vi "dms-main-train-2.vi"() -> ()   [LabVIEW 2015]
uses:
  states-enum.ctl
  <vilib>/platform/TimedLoop/XDataNode/XDataNode.xnode
  <vilib>/Platform/TimedLoop/XDataNode/nitl_modes.ctl
  <vilib>/Platform/TimedLoop/XDataNode/XDNodeRunTimeDep.lvlib
  <vilib>/Platform/TimedLoop/XDataNode/wakeup.ctl
  <vilib>/Platform/TimedLoop/XDataNode/timing_clust.ctl
  Device/Methods/Speaker-Play.vi
  Rack/Methods/Rack-Refresh.vi
  Device/Methods/Lickometer-Read.vi
  Device/Methods/Valve-Init.vi
  Device/Methods/Juicer-Init.vi
  Device/Methods/Speaker-Init.vi
  Rack/Methods/Rack-Start.vi
  Rack/Methods/Rack-Config.vi
  Device/Methods/Lickometer-Init.vi
  Rack/Methods/Rack-Init.vi
  Device/Methods/Valve-Pulse.vi
  <vilib>/Utility/file.llb/Read Delimited Spreadsheet (I64).vi
  Device/Methods/Lickometer-Stop.vi
  Rack/Methods/Rack-Stop.vi
  Rack/Typedefs/OutputRequest.ctl
  Rack/Typedefs/OutputRequest refnum.ctl
  Rack/Methods/Port drivers/DigitalInput-DataCluster.ctl
  Rack/Typedefs/InputData cluster.ctl
  Device/Typedefs/Lickometer.ctl
  Device/Typedefs/Speaker.ctl
  Device/Typedefs/Juicer.ctl
  Device/Typedefs/Valve.ctl
panel:
  out "InputData 3":T1
  out "InputData 2":T1
  in  "stop":bool
  out "Acc":dbl
  out "Time":dbl format="%#.0f"
  out "Trials":string
  out "Reward Dispensed (uL)":string
  out "Licks":string
  out "CR":string
  out "Miss":string
  out "FA":string
  out "Hits":string
  out "Current State":string
  out "Time Elapsed":dbl format="%<%H:%M:%S>t"
  in  "Tab Control":enum32{"Required", "Optional", "Devices"}(tab)
  in  "Tone Pairs":u16(ring) items=["1: 3000 Hz, 12000 Hz", "2: 5800 Hz, 5000 Hz", "3: 5000 Hz, 10000 Hz", "4: 8000 Hz, 15000 Hz"]
  in  "Max Time (s)":dbl=3600.0
  in  "Number of trials":string(combo)="500"
  in  "Max number of \nconsecutive trials":string(combo)="3"
  in  "Animal Name":string="Mouse"
  in  "Reward Vol. (uL)":dbl=5.0
  in  "Sequence Directory":path=path "C:/Users/SiapasLab/Desktop/git/wheatley"
  in  "Assay Description":string="Auditory delayed match to sample"
  in  "Recording Location":string="BI Room 146"
  in  "Trial delay (ms)":dbl=1500.0
  in  "Punish Time (s)":dbl
  in  "Trial window (ms)":dbl=1000.0
  in  "ITI lower (s)":dbl=10.0
  in  "ITI upper (s)":dbl=10.0
  in  "Min Licks":i32=1 min=1
  in  "Data Saving Directory":path=path "\\\\CA1-17\\ld8007/anesthesia/data"
  in  "Lickometer":T3={"Settings"={"Min lick duration"=1, "Port name"="bnc_panel.p0.3", "Port index"=0}, "Lick"=FALSE, "Debouncing"={"Semaphore"=refnum, "Lick start"=0}, "OutputRequest event ref"=refnum, "InputData reference"=refnum, "Active hi?"=FALSE}
  out "InputData":T1
  in  "Speaker":T6={"Settings"={"Portname"="BNC_Panel.ao0", "Index"=0, "Timestamp portname"="BNC_Panel.P0.0"}, "OutputRequest event ref"=refnum, "InputData reference"=refnum}
  in  "Juicer":T7={"Mode"=enum."Juice/reward", "Settings"={"Bleed #1 port index"=1, "Bleed #1 port name"="juicer.bleed1", "Bleed #2 port name"="juicer.bleed2", "Bleed #2 port index"=2, "Flush port name"="juicer.flush", "Flush port index"=3, "Purge port name"="juicer.purge", "Purge port index"=0, "Timestamp port name"="dsub_panel.p9.7"}, "OutputRequest event ref"=refnum, "InputData reference"=refnum}
  in  "Valve":T8={"Settings"={"Timestamp port name"="BNC_panel.P0.0", "Port name"="BNC_panel.P0.1", "Port index"=4}, "OutputRequest event ref"=refnum, "InputData reference"=refnum, "Default length (ms)"=100}
  # "Auditory delayed match to sample task (DMS)"
  # "(must be on same NI card)"
  # "(must be on same NI card)"
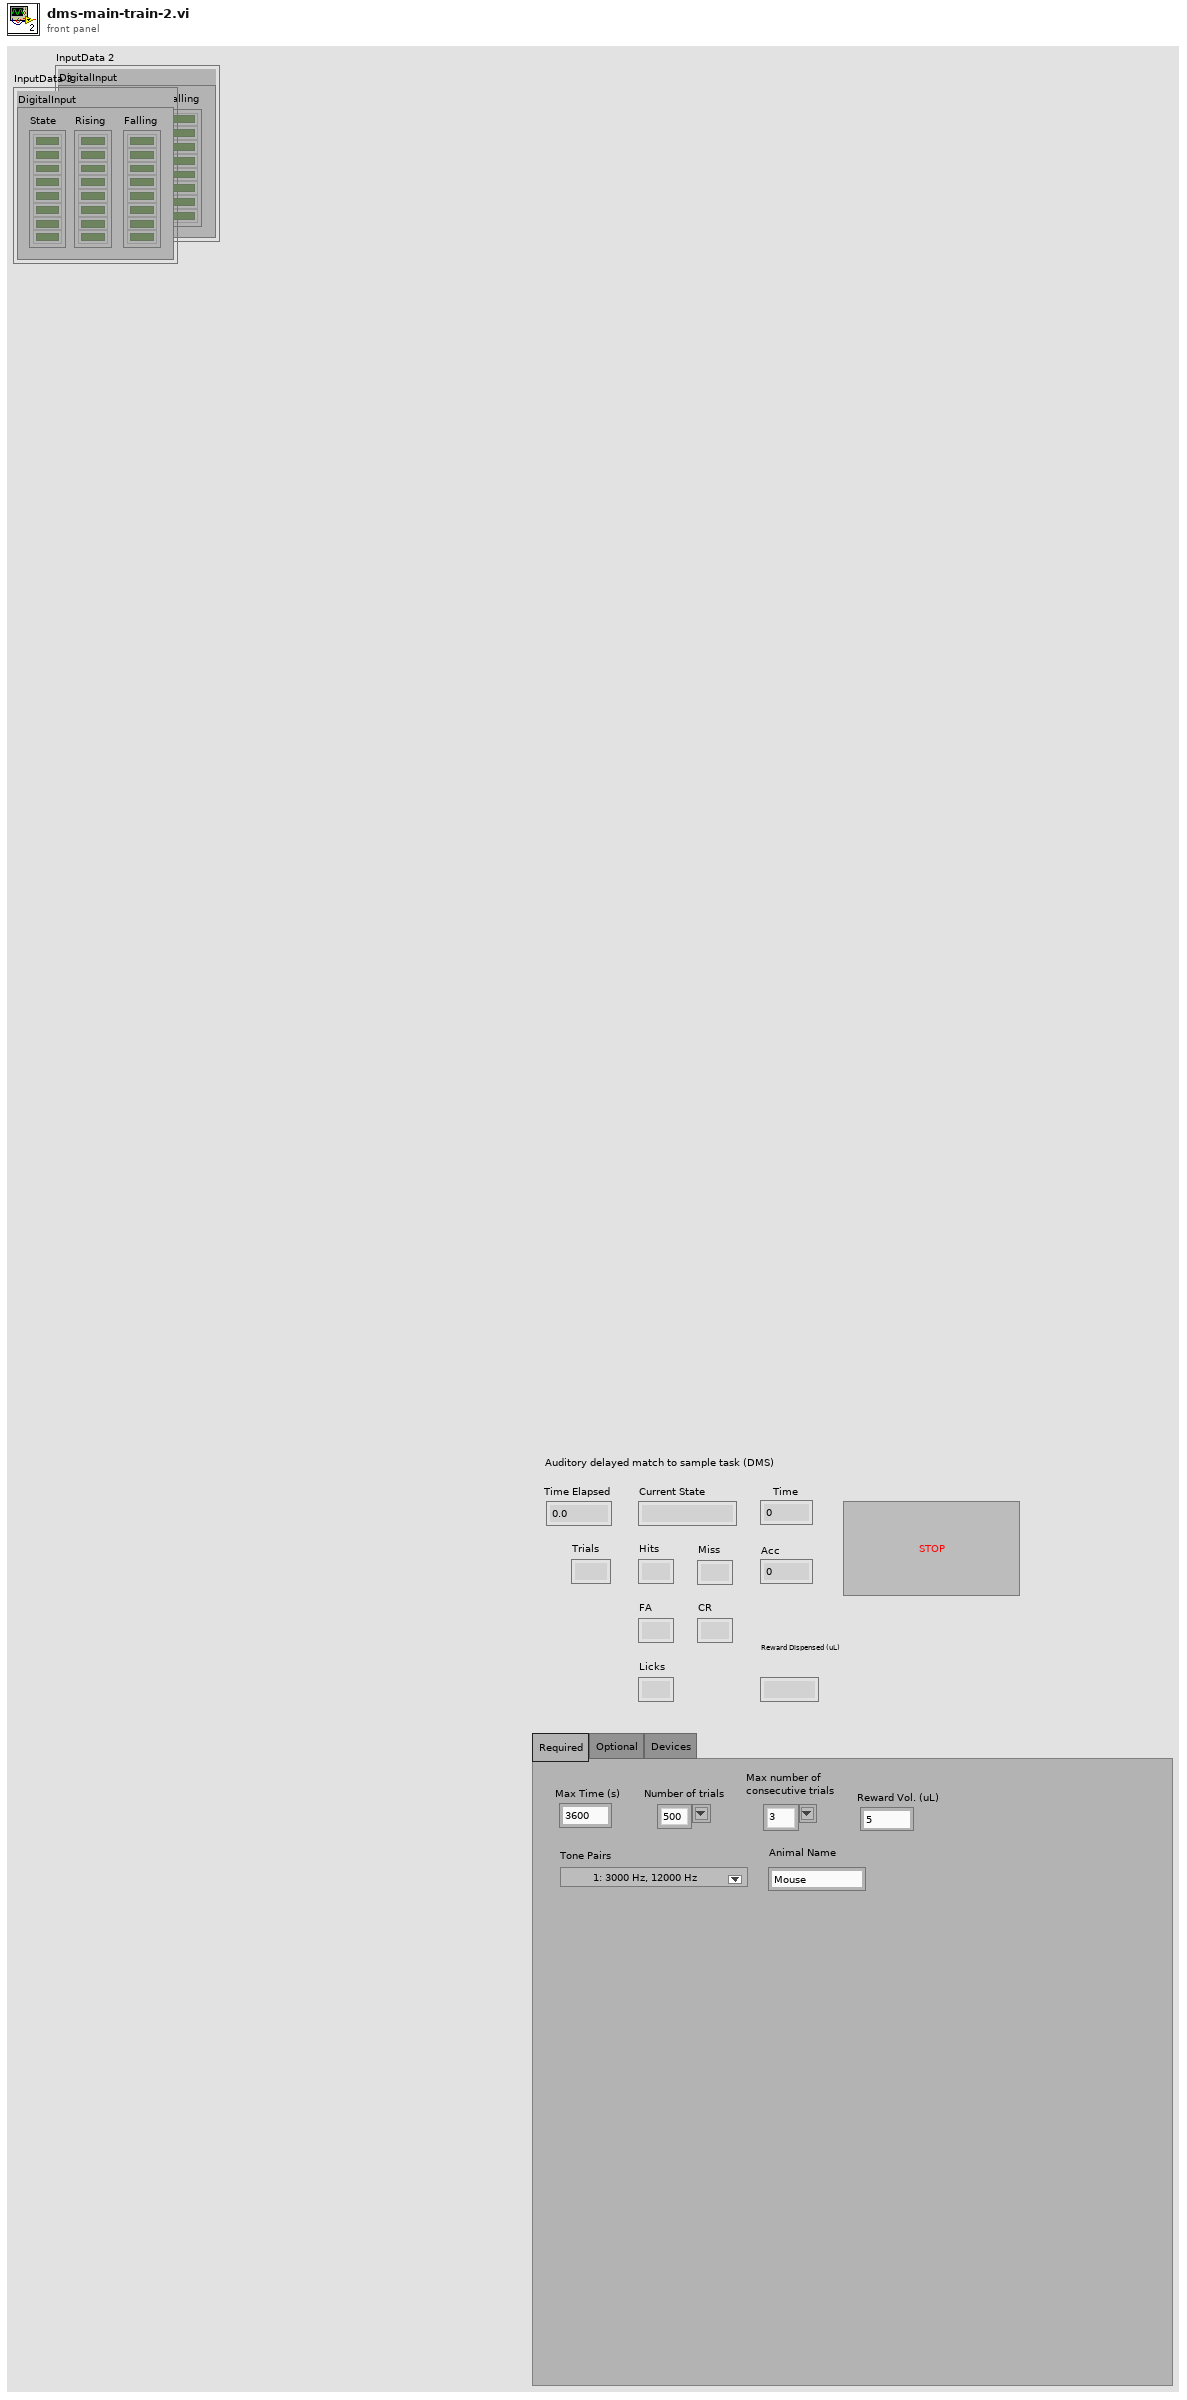
[diagram p1: front panel]
types:
  T1 = typedef "InputData cluster.ctl" = cluster{"DigitalInput":T2}
  T2 = typedef "DigitalInput-DataCluster.ctl" = cluster{"Falling":bool[], "Rising":bool[], "State":bool[]}
  T3 = typedef "Lickometer.ctl" = cluster{"Settings":cluster{"Min lick duration":u32, "Port name":string, "Port index":i32}, "Lick":bool, "Debouncing":cluster{"Semaphore":T4, "Lick start":u32}, "OutputRequest event ref":T5, "InputData reference":refnum<vi>, "Active hi?":bool}
  T4 = typedef "Semaphore RefNum" = refnum<k1>
  T5 = typedef "OutputRequest refnum.ctl" = refnum<user-event>
  T6 = typedef "Speaker.ctl" = cluster{"Settings":cluster{"Portname":string, "Index":i32, "Timestamp portname":string}, "OutputRequest event ref":T5, "InputData reference":refnum<vi>}
  T7 = typedef "Juicer.ctl" = cluster{"Mode":enum16{"Off", "Juice/reward", "Water flush", "Air purge"}, "Settings":cluster{"Bleed #1 port index":i32, "Bleed #1 port name":string, "Bleed #2 port name":string, "Bleed #2 port index":i32, "Flush port name":string, "Flush port index":i32, "Purge port name":string, "Purge port index":i32, "Timestamp port name":string}, "OutputRequest event ref":T5, "InputData reference":refnum<vi>}
  T8 = typedef "Valve.ctl" = cluster{"Settings":cluster{"Timestamp port name":string, "Port name":string, "Port index":i32}, "OutputRequest event ref":T5, "InputData reference":refnum<vi>, "Default length (ms)":i32}
  T9 = typedef "states-enum.ctl" = enum16{"ITI", "Trial", "Stop"}
  T10 = typedef "Rack driver configuration cluster.ctl" = cluster{"DigitalInput":T11, "DigitalOutput":T12, "FileOutput":T13, "AnalogOutput":T14, "DataSocketOutput":T15}
  T11 = typedef "DigitalInput-Configuration.ctl" = cluster{"Lines":tag[], "Refresh period (ms)":u32}
  T12 = typedef "DigitalOutput-Configuration.ctl" = cluster{"Output Lines":tag[], "DO timestamp lines":tag[], "Timestamp lines":tag[]}
  T13 = typedef "FileOutput-Configuration.ctl" = cluster{"Logfile path":path}
  T14 = typedef "AnalogOutput-Configuration.ctl" = cluster{"Output Lines":tag[], "AO timestamp lines":tag[]}
  T15 = typedef "DataSocketOutput-Configuration.ctl" = cluster{"DataSocket URL":string}
  T16 = cluster{"ITI upper (s)":dbl, "ITI lower (s)":dbl, "Punish Time (s)":dbl, "Trial window (ms)":dbl, "Trial delay (ms)":dbl, "Max Time (s)":dbl, "Min Licks":i32, "Reward Vol. (uL)":dbl, "Tone 1":i32, "Tone 2":i32}
  T17 = cluster{"appended path":path, "relative seconds":dbl, "Current Trial Index":i32, "Accuracy":dbl, "Hits":i32, "Miss":i32, "False Alarm":i32, "Correct Rejection":i32, "Licks":i32, "Reward Dispensed":dbl, "Punish ITI":bool, "Next Trial":i32}
  T18 = typedef "XDNodeRunTimeDep.lvlib/timing_clust.ctl" = cluster{"Expected End [f-1]":u64, "Actual End [f-1]":u64, "Finished Late? [f-1]":bool, "Expected End [i-1]":u64, "Actual End [i-1]":u64, "Finished Late? [i-1]":bool, "Expected Start [i]":u64, "Actual Start [i]":u64, "Expected Start [f]":u64, "Actual Start [f]":u64, "Source Name":string, "Structure Name":string, "Period":i64, "Deadline":i64, "Offset":i64, "Start":i64, "Priority":i32, "Timeout":i32, "Mode":T19, "Wakeup Reason":T20, "Error":errorcluster, "Source Type":string, "Secondary Source Type":string, "Global End Time":u64, "Global Start Time":u64, "Frame Duration":u64, "Iteration Duration":u64, "Assigned CPU":i32, "I/O Scan Engine Mode":u32}
  T19 = typedef "XDNodeRunTimeDep.lvlib/nitl_modes.ctl" = enum32{"No Change", "Process missed periods, maintain original phase", "Discard missed periods, maintain original phase", "Process missed periods, ignore original phase", "Discard missed periods, ignore original phase"}
  T20 = typedef "XDNodeRunTimeDep.lvlib/wakeup.ctl" = enum32{"Normal", "Aborted", "Asynchronous wakeup", "Timing source error", "Timed loop error", "Timeout"}
  T21 = cluster{"Trial Hit":bool, "Trial Miss":bool, "Trial FA":bool, "Trial CR":bool, "Skip Receiving":bool}
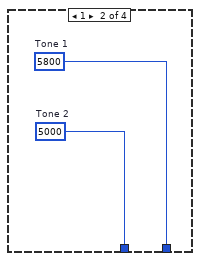
[diagram p2: hidden frame]
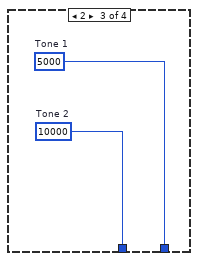
[diagram p3: hidden frame]
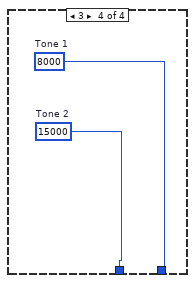
[diagram p4: hidden frame]
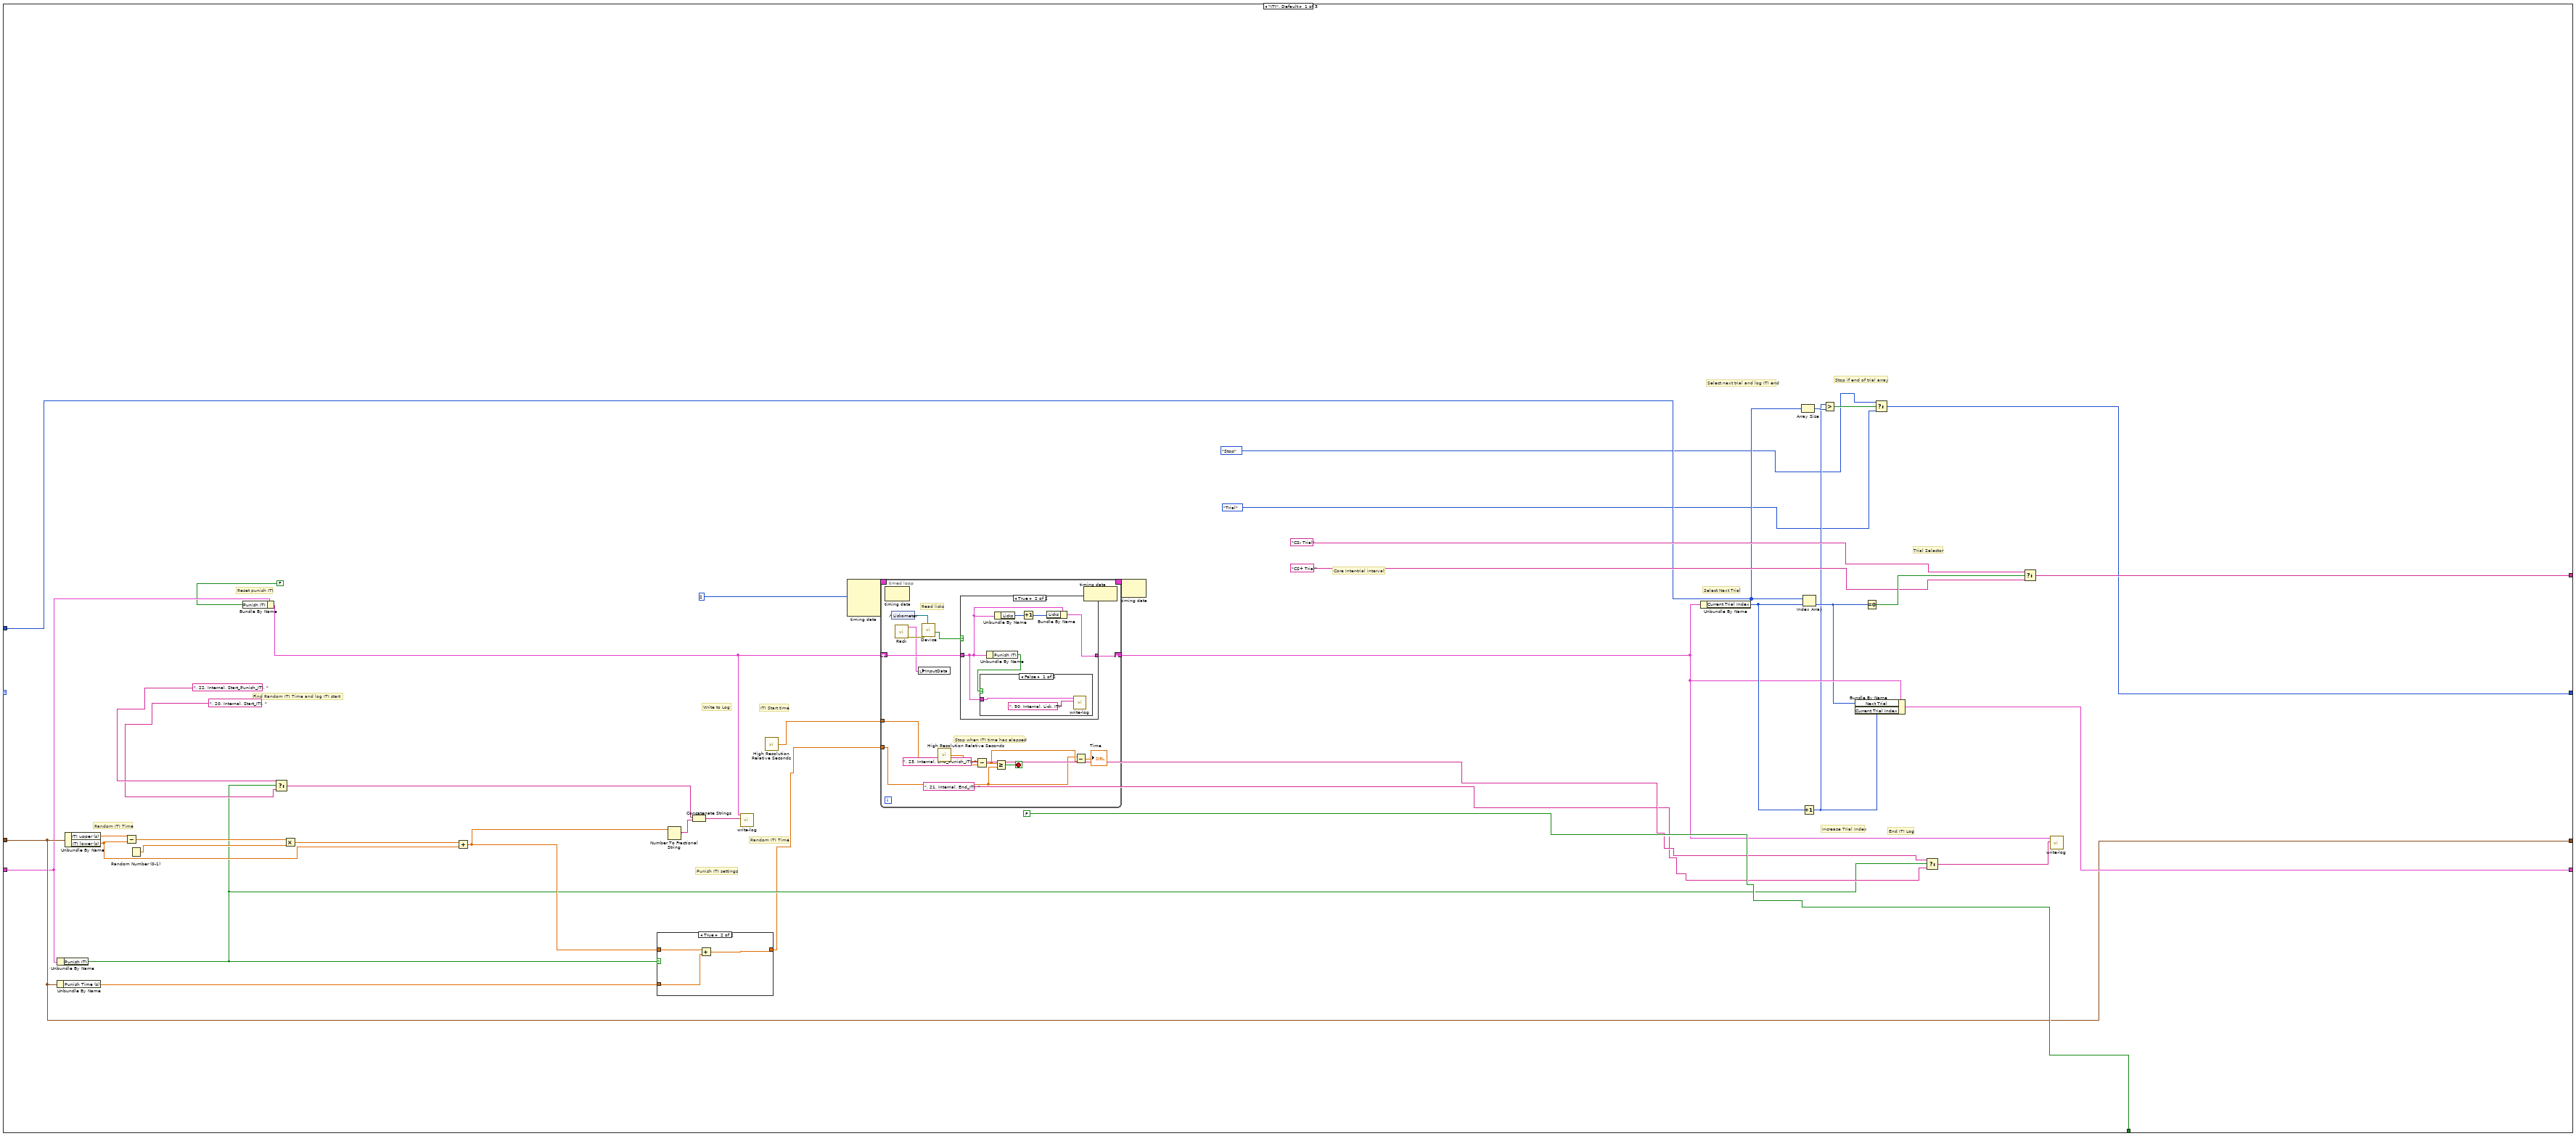
[diagram p6: hidden frame]
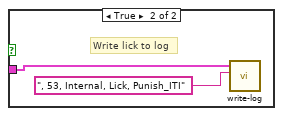
[diagram p8: hidden frame]
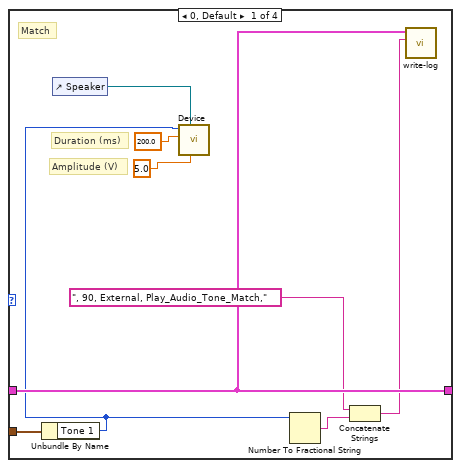
[diagram p11: hidden frame]
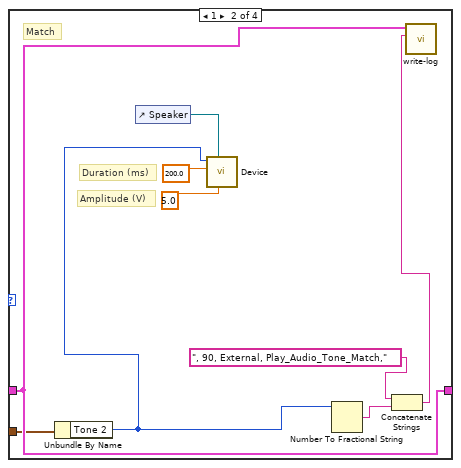
[diagram p12: hidden frame]
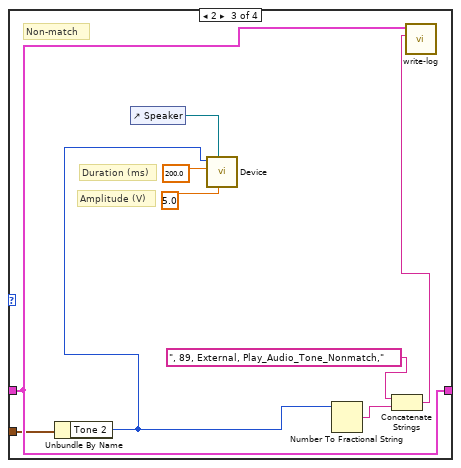
[diagram p13: hidden frame]
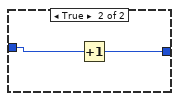
[diagram p14: hidden frame]
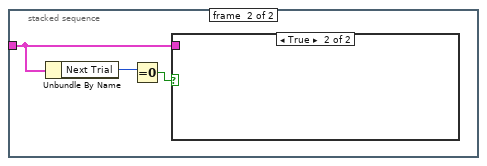
[diagram p16: hidden frame]
diagram:
  w141 = 0  # Next Trial
  w142 = FALSE  # Punish ITI
  w151 = 0.0  # Reward Dispensed
  w152 = 0  # Licks
  w153 = 0  # Correct Rejection
  w154 = 0  # False Alarm
  w157 = 0.0  # Accuracy
  w155 = 0  # Miss
  w156 = 0  # Hits
  w158 = 0  # Current Trial Index
  # "Create directory"
  # "Lickometer"
  # "Lickometer"
  # "Devices"
  # "Tone Pair Interpretation"
  # "Exit Logging"
  # "Front Panel Logging"
  # "CS+\nDelay lick: Miss\nReception lick: Hit\nNo lick: Miss\n\nCS-\nDelay lick: False alarm\nReception lick: False alarm\nNo lick: Correct reject"
  # "Start time"
  # "Internal Variables"
  # "External variables from Front Panel"
  # "External variable cluster"
  # "Internal variable cluster"
  # "State enum"
  # "Trial shift register"
  # "State machine"
  # "Front Panel Elements"
  # "Write trial sequence to log"
  # "Human readable time"
  # "End of header delimiter"
  # "Start Time"
  # "Environment"
  # "Schedule"
  # "Initialize data logger"
  # "Random sequence selection"
  # "Read in entire .csv"
  # "Load pre-generated sequences"
  n1 = Format Date/Time String(time format string (%c)="%Y-%m-%d-%H-%M-%S") -> (date/time string=w4:string)  [unwired: 2 in]
  n2 = case shown="0, Default" "Tone Pairs" {
    tunnel: [w224 w225 w227 w229] -> w39
    tunnel: [w223 w226 w228 w230] -> w40
    frame 0, Default {
      w224 = 12000  # Tone 2
      w223 = 3000  # Tone 1
    }
    frame 1 {
      w225 = 5000  # Tone 2
      w226 = 5800  # Tone 1
    }
    frame 2 {
      w227 = 10000  # Tone 2
      w228 = 5000  # Tone 1
    }
    frame 3 {
      w229 = 15000  # Tone 2
      w230 = 8000  # Tone 1
    }
  }
  n3 = Build Path(base path="Data Saving Directory", name or relative path=w4) -> (appended path=w2:path)
  n4 = Create Folder(path (use dialog)=w2) -> (created path=w1:path)  [unwired: 2 in, 2 out]
  n5 = control-ref of="InputData"() -> (w13:refnum<vi>)
  n6 = Build Path(base path=w1, name or relative path="data.txt") -> (appended path=w148:path)
  n7 = call-poly "Rack.vi"() -> ("error out"=w7:errorcluster, "OutputRequest\nevent ref"=w8:T5)  [unwired: 10 in]
  n8 = control-ref of="Juicer"() -> (w6:refnum<vi>)
  n9 = Path To String(path="Sequence Directory") -> (string=w96:string)
  n10 = call-poly "Device.vi"("Device reference"=w6, "error in (no error)"=w7, "OutputRequest event ref"=w8, "InputData reference"=w13) -> ("error out"=w10:errorcluster, "OutputRequest (dup)"=w15:T5, "InputData (dup)"=w12:refnum<vi>)  [unwired: 5 in]
  n11 = control-ref of="Valve"() -> (w5:refnum<vi>)
  n12 = Concatenate Strings(w96, "\\sequences\\seq_n_", "Number of trials", "_k_" ("string"), "Max number of \nconsecutive trials", "_m_2.csv" ("string")) -> (w214:string)
  n13 = call-poly "Device.vi"("Device reference"=w5, "error in (no error)"=w10, "OutputRequest event ref"=w15, "InputData reference"=w12) -> ("error out"=w9:errorcluster, "OutputRequest (dup)"=w14:T5, "InputData (dup)"=w11:refnum<vi>)  [unwired: 5 in]
  n14 = String To Path(string=w214) -> (path=w215:path)
  n15 = control-ref of="Speaker"() -> (w16:refnum<vi>)
  n16 = Concatenate Strings("Schedule," ("string"), "Assay Description", "\r\n") -> (w205:string)
  n17 = call-poly "Device.vi"("Device reference"=w16, "error in (no error)"=w9, "OutputRequest event ref"=w14, "InputData reference"=w11) -> ("error out"=w18:errorcluster, "OutputRequest (dup)"=w19:T5, "InputData (dup)"=w17:refnum<vi>)  [unwired: 5 in]
  n18 = Concatenate Strings("Path," ("string"), w96, "\r\n") -> (w99:string)
  n19 = call-poly <vilib>:"Read Delimited Spreadsheet.vi"("file path (dialog if empty)"=w215, "number of rows (all:-1)"=-1, "delimiter (\\t)"="," ("delimiter (\\t)")) -> ("all rows"=w209:i64[][])  [unwired: 7 in, 5 out]
  n20 = Write to Text File(file (use dialog)=w148, text=w205) -> (refnum out=w207:refnum<file>)  [unwired: 2 in, 2 out]
  n21 = control-ref of="Lickometer"() -> (w23:refnum<vi>)
  n22 = call-poly "Device.vi"("Device reference"=w23, "error in (no error)"=w18, "OutputRequest event ref"=w19, "InputData reference"=w17) -> ("error out"=w28:errorcluster, "OutputRequest (dup)"=w25:T5)  [unwired: 5 in, 1 out]
  n23 = Concatenate Strings("Environment," ("string"), "Recording Location", "\r\n") -> (w201:string)
  n24 = Array Size(array=w209) -> (size(s)=w213:i32[])
  n25 = Write to Text File(file (use dialog)=w207, text=w201) -> (refnum out=w101:refnum<file>)  [unwired: 2 in, 2 out]
  n26 = Format Date/Time String() -> (date/time string=w175:string)  [unwired: 3 in]
  n27 = call-poly "Rack.vi"("error in (no error)"=w28) -> ("error out"=w27:errorcluster, "Configuration"=w26:T10)  [unwired: 9 in]
  n28 = Index Array(array=w213, index=0) -> (element=w211:i32)
  n29 = Random Number (0-1)() -> (number: 0 to 1=w220:dbl)
  n30 = Write to Text File(file (use dialog)=w101, text=w99) -> (refnum out=w100:refnum<file>)  [unwired: 2 in, 2 out]
  n31 = Decrement(x=w211) -> (x-1=w210:i32)
  n32 = call-poly "Rack.vi"("error in (no error)"=w27, "OutputRequest event ref"=w25, "Configuration"=w26) -> ("OutputRequest event ref (dup)"=w21:T5)  [unwired: 7 in, 1 out]
  n33 = Multiply(x=w220, y=w210) -> (x*y=w219:dbl)
  n34 = Concatenate Strings("Time," ("string"), w175, "\r\n") -> (w197:string)
  n35 = To Long Integer(number=w219) -> (32bit integer=w208:i32)
  n36 = Write to Text File(file (use dialog)=w100, text=w197) -> (refnum out=w196:refnum<file>)  [unwired: 2 in, 2 out]
  n37 = call <vilib>:"High Resolution Relative Seconds.vi"() -> ("relative seconds"=w160:dbl)
  n38 = Index Array(array=w209, index (row)=w208) -> (element=w150:i64[])  [unwired: 1 in]
  n39 = Bundle("ITI upper (s)"="ITI upper (s)", "ITI lower (s)"="ITI lower (s)", "Punish Time (s)"="Punish Time (s)", "Trial window (ms)"="Trial window (ms)", "Trial delay (ms)"="Trial delay (ms)", "Max Time (s)"="Max Time (s)", "Min Licks"="Min Licks", "Reward Vol. (uL)"="Reward Vol. (uL)", "Tone 1"=w40, "Tone 2"=w39) -> (w135:T16)  [unwired: 1 in]
  n40 = Concatenate Strings("Animal," ("string"), "Animal Name", "\r\n") -> (w193:string)
  n41 = Unbundle By Name(w135) -> ("Max Time (s)"=w134:dbl, "Trial delay (ms)"=w133:dbl, "Trial window (ms)"=w132:dbl, "ITI lower (s)"=w131:dbl, "ITI upper (s)"=w130:dbl, "Punish Time (s)"=w129:dbl, "Min Licks"=w52:i32, "Reward Vol. (uL)"=w44:dbl, "Tone 1"=w32:i32, "Tone 2"=w31:i32)
  n42 = Write to Text File(file (use dialog)=w196, text=w193) -> (refnum out=w185:refnum<file>)  [unwired: 2 in, 2 out]
  n43 = Bundle("appended path"=w148, "relative seconds"=w160, "Current Trial Index"=w158, "Accuracy"=w157, "Hits"=w156, "Miss"=w155, "False Alarm"=w154, "Correct Rejection"=w153, "Licks"=w152, "Reward Dispensed"=w151, "Punish ITI"=w142, "Next Trial"=w141) -> (w159:T17)  [unwired: 1 in]
  n44 = for {
    N -> [w232]
    shift-right: [w236] -> w140
    shift-left: " " -> [w237]
    tunnel: w150 -> [w239] mode=indexing
    i -> [w235]
    n45 = Decrement(x=w232) -> (x-1=w231:i32)
    n46 = Equal?(x=w231, y=w235) -> (x = y?=w234:bool)
    n47 = Number To Decimal String(number=w239) -> (decimal integer string=w238:string)  [unwired: 1 in]
    n48 = case shown="False" w234 {
      tunnel: [", " ("string") "" ("string")] -> w233
      frame False {
      }
      frame True {
      }
    }
    n49 = Concatenate Strings(w237, w238, w233) -> (w236:string)
  }
  n50 = Concatenate Strings("Trials," ("string"), "Number of trials", "\r\n") -> (w189:string)
  n51 = Write to Text File(file (use dialog)=w185, text=w189) -> (refnum out=w184:refnum<file>)  [unwired: 2 in, 2 out]
  n52 = Number To Fractional String(number=w32) -> (F-format string=w33:string)  [unwired: 3 in]
  n53 = Number To Fractional String(number=w44) -> (F-format string=w43:string)  [unwired: 3 in]
  n54 = Number To Fractional String(number=w31) -> (F-format string=w34:string)  [unwired: 3 in]
  n55 = Number To Fractional String(number=w134) -> (F-format string=w128:string)  [unwired: 3 in]
  n56 = Number To Fractional String(number=w129) -> (F-format string=w116:string)  [unwired: 3 in]
  n57 = Number To Fractional String(number=w52) -> (F-format string=w51:string)  [unwired: 3 in]
  n58 = Number To Fractional String(number=w133) -> (F-format string=w125:string)  [unwired: 3 in]
  n59 = Number To Fractional String(number=w132) -> (F-format string=w122:string)  [unwired: 3 in]
  n60 = Number To Fractional String(number=w131) -> (F-format string=w121:string)  [unwired: 3 in]
  n61 = Number To Fractional String(number=w130) -> (F-format string=w119:string)  [unwired: 3 in]
  n62 = Concatenate Strings("Max_Time_s," ("string"), w128, "\r\n") -> (w110:string)
  n63 = Concatenate Strings("Consecutive_Trials," ("string"), "Max number of \nconsecutive trials", "\r\n") -> (w186:string)
  n64 = Concatenate Strings("CS+_Tone," ("string"), w33, "\r\n") -> (w30:string)
  n65 = Concatenate Strings("Min_Licks," ("string"), w51, "\r\n") -> (w48:string)
  n66 = Concatenate Strings("Reward_Volume," ("string"), w43, "\r\n") -> (w42:string)
  n67 = Concatenate Strings("CS-_Tone," ("string"), w34, "\r\n") -> (w29:string)
  n68 = Concatenate Strings("Delay_Window_ms," ("string"), w125, "\r\n") -> (w109:string)
  n69 = Concatenate Strings("ITI_Lower_s," ("string"), w121, "\r\n") -> (w107:string)
  n70 = Concatenate Strings("Reception_Window_ms," ("string"), w122, "\r\n") -> (w108:string)
  n71 = Concatenate Strings("ITI_Upper_s," ("string"), w119, "\r\n") -> (w106:string)
  n72 = Concatenate Strings("Punish_Time_s," ("string"), w116, "\r\n") -> (w105:string)
  n73 = Write to Text File(file (use dialog)=w184, text=w186) -> (refnum out=w104:refnum<file>)  [unwired: 2 in, 2 out]
  n74 = while {
    shift-right: [w275] -> _
    shift-left: states-enum."ITI" -> [w252]
    shift-right: [w251] -> _
    shift-left: w135 -> [w267]
    shift-right: [w266] -> w60
    shift-left: w159 -> [w246]
    tunnel: w150 -> [w269]
    tunnel: w21 -> [w245]
    tunnel: [w245] -> w20
    stop <- w247 stop-if-true
    # "State enum"
    # "Internal variable cluster"
    # "External variable cluster"
    # "Update front panel"
    # "Update front panel"
    # "Wait for current state to finish before ending session"
    n75 = case shown="\"Trial\"" w252 {
      tunnel: [w294 states-enum."ITI" states-enum."Stop"] -> w275
      tunnel: [FALSE FALSE TRUE] -> w271
      tunnel: w269 -> [w299 _ _]
      tunnel: [w303 w402 "Stop"] -> w268
      tunnel: w267 -> [w302 w355 w749]
      tunnel: [w308 w368 w745] -> w266
      tunnel: w246 -> [w293 w371 w745]
      tunnel: [w302 w355 w749] -> w251
      frame "ITI", Default {
        # "Reset punish ITI"
        # "Stop if end of trial array"
        # "Punish ITI settings"
        # "Select next trial and log ITI end"
        # "Trial Selector"
        # "Increase Trial Index"
        # "Select Next Trial"
        # "End ITI Log"
        # "ITI Start time"
        # "Core Inter-trial interval"
        # "Find Random ITI Time and log ITI start"
        # "Random ITI Time"
        # "Write to Log"
        # "Random ITI Time"
        n76 = Unbundle By Name(w302) -> ("Punish Time (s)"=w301:dbl)
        n77 = Unbundle By Name(w293) -> ("Punish ITI"=w284:bool)
        n78 = Unbundle By Name(w302) -> ("ITI upper (s)"=w311:dbl, "ITI lower (s)"=w315:dbl)
        n79 = Subtract(x=w311, y=w315) -> (x-y=w312:dbl)
        n80 = Random Number (0-1)() -> (number: 0 to 1=w313:dbl)
        n81 = Bundle By Name(cluster=w293, "Punish ITI"=FALSE) -> (w292:T17)
        n82 = Select(t=", 22, Internal, Start_Punish_ITI, " ("text"), s=w284, f=", 20, Internal, Start_ITI, " ("text")) -> (s? t:f=w288:string)
        n83 = Multiply(x=w312, y=w313) -> (x*y=w314:dbl)
        n84 = Add(x=w314, y=w315) -> (x+y=w300:dbl)
        n85 = case shown="True" w284 {
          tunnel: w300 -> [w347 w350]
          tunnel: [w347 w349] -> w282
          tunnel: w301 -> [_ w348]
          frame False {
          }
          frame True {
            n86 = Add(x=w350, y=w348) -> (x+y=w349:dbl)
          }
        }
        n87 = Number To Fractional String(number=w300) -> (F-format string=w317:string)  [unwired: 3 in]
        n88 = Concatenate Strings(w288, w317) -> (w316:string)
        n89 = call "write-log.vi"("Write Text"=w316, "Internal Cluster"=w292) -> ()  [unwired: 10 in]
        n90 = call <vilib>:"High Resolution Relative Seconds.vi"() -> ("relative seconds"=w283:dbl)
        n91 = node-c288(i64 2 ("Period")) -> (w281:T18)  [unwired: 3 in]
        n92 = timed-loop {
          tunnel: w282 -> [w323]
          tunnel: w283 -> [w324]
          shift-right: [w327] -> w309
          shift-left: w292 -> [w328]
          timing: w281 -> [_]
          timing-out: [_] -> w280
          stop <- w329 stop-if-true
          # "Read licks"
          # "Stop when ITI time has elapsed"
          n93 = node-c288() -> ()  [unwired: 1 in, 1 out]
          n94 = control-ref of="Lickometer"() -> (w322:refnum<vi>)
          n95 = call-poly "Rack.vi"() -> ("error out"=w321:errorcluster, "Data Cluster"=w319:T1)  [unwired: 10 in]
          n96 = local write "InputData"(w319) -> ()
          n97 = call-poly "Device.vi"("Device reference"=w322, "error in (no error)"=w321) -> ("Lick start?"=w320:bool)  [unwired: 7 in, 2 out]
          n98 = call <vilib>:"High Resolution Relative Seconds.vi"() -> ("relative seconds"=w330:dbl)
          n99 = case shown="True" w320 {
            tunnel: w328 -> [w333 w334]
            tunnel: [w333 w336] -> w327
            frame False {
            }
            frame True {
              n100 = Unbundle By Name(w334) -> ("Punish ITI"=w335:bool)
              n101 = case shown="False" w335 {
                tunnel: w334 -> [w340 w341]
                frame False {
                  n102 = call "write-log.vi"("Write Text"=", 50, Internal, Lick, ITI" ("text"), "Internal Cluster"=w340) -> ()  [unwired: 10 in]
                }
                frame True {
                  # "Write lick to log"
                  n103 = call "write-log.vi"("Write Text"=", 53, Internal, Lick, Punish_ITI" ("text"), "Internal Cluster"=w341) -> ()  [unwired: 10 in]
                }
              }
              n104 = Unbundle By Name(w334) -> ("Licks"=w338:i32)
              n105 = Increment(x=w338) -> (x+1=w337:i32)
              n106 = Bundle By Name(cluster=w334, "Licks"=w337) -> (w336:T17)
            }
          }
          n107 = Subtract(x=w330, y=w324) -> (x-y=w325:dbl)
          n108 = Greater Or Equal?(x=w325, y=w323) -> (x >= y?=w329:bool)
          n109 = Subtract(x=w323, y=w325) -> (x-y=→"Time":dbl)
          n110 = node-c288() -> ()  [unwired: 1 in, 1 out]
        }
        n111 = node-c288(w280) -> ()  [unwired: 1 out]
        n112 = Unbundle By Name(w309) -> ("Current Trial Index"=w310:i32)
        n113 = Array Size(array=w299) -> (size(s)=w298:i32)
        n114 = Increment(x=w310) -> (x+1=w297:i32)
        n115 = Index Array(array=w299, index=w310) -> (element=w307:i64)
        n116 = Greater?(x=w297, y=w298) -> (0:w296:bool)
        n117 = Bundle By Name(cluster=w309, "Next Trial"=w307, "Current Trial Index"=w297) -> (w308:T17)
        n118 = Equal To 0?(x=w307) -> (x = 0?=w306:bool)
        n119 = Select(t=states-enum."Stop", s=w296, f=states-enum."Trial") -> (s? t:f=w294:T9)
        n120 = Select(t=", 23, Internal, End_Punish_ITI, " ("text"), s=w284, f=", 21, Internal, End_ITI, " ("text")) -> (s? t:f=w287:string)
        n121 = Select(t="CS- Trial", s=w306, f="CS+ Trial") -> (s? t:f=w303:string)
        n122 = call "write-log.vi"("Write Text"=w287, "Internal Cluster"=w309) -> ()  [unwired: 10 in]
      }
      frame "Trial" {
        w373 = 0  # Current Number Reception Licks
        w374 = 0  # Current Number Delay Licks
        w376 = FALSE  # Skip Receiving
        # "Only reward hit"
        # "Log metrics"
        # "Trial Window Log"
        # "Dispense reward"
        # "Enable punishment if FA or CR"
        # "Accuracy"
        # "Update metrics using local cluster"
        # "S+ No Lick - Miss\nS- No Lick - Correct Reject"
        # "Convert to s"
        # "Trial Reception Window"
        # "Convert to s"
        # "Trial Start Time"
        # "Trial Delay"
        n123 = node-c288(i64 2 ("Period")) -> (w366:T18)  [unwired: 3 in]
        n124 = Unbundle By Name(w371) -> ("Next Trial"=w351:i32)
        n125 = case shown="3" w351 {
          tunnel: w371 -> [w709 w711 w713 w715]
          tunnel: [w709 w711 w713 w715] -> w370
          frame 0, Default {
            # "Match"
            n126 = call "write-log.vi"("Write Text"=", 95, Internal, Start_Match_Trial, " ("text"), "Internal Cluster"=w709) -> ()  [unwired: 10 in]
          }
          frame 1 {
            # "Match"
            n127 = call "write-log.vi"("Write Text"=", 95, Internal, Start_Match_Trial, " ("text"), "Internal Cluster"=w711) -> ()  [unwired: 10 in]
          }
          frame 2 {
            # "Non-match"
            n128 = call "write-log.vi"("Write Text"=", 96, Internal, Start_Nonmatch_Trial, " ("text"), "Internal Cluster"=w713) -> ()  [unwired: 10 in]
          }
          frame 3 {
            # "Nonmatch"
            n129 = call "write-log.vi"("Write Text"=", 96, Internal, Start_Nonmatch_Trial, " ("text"), "Internal Cluster"=w715) -> ()  [unwired: 10 in]
          }
        }
        n130 = timed-loop {
          tunnel: w370 -> [w646]
          tunnel: [w640] -> w430
          tunnel: w355 -> [w645]
          timing: w366 -> [_]
          timing-out: [_] -> w365
          stop <- TRUE stop-if-true
          # "Read Speaker Lick"
          # "Play Sound While Loop"
          n131 = node-c288() -> ()  [unwired: 1 in, 1 out]
          n132 = Unbundle By Name(w646) -> ("Next Trial"=w638:i32)
          n133 = case shown="1" w638 {
            tunnel: w646 -> [w664 w673 w682 w691]
            tunnel: [w664 w673 w682 w691] -> w641
            tunnel: w645 -> [w663 w669 w678 w687]
            frame 0, Default {
              # "Duration (ms)"
              # "Amplitude (V)"
              # "Match"
              n134 = Unbundle By Name(w663) -> ("Tone 1"=w656:i32)
              n135 = control-ref of="Speaker"() -> (w657:refnum<vi>)
              n136 = call-poly "Device.vi"("Amplitude (V)"=5.0, "Device reference"=w657, "Duration (ms)"=200.0, "Frequency (Hz)"=w656) -> ()  [unwired: 7 in, 1 out]
              n137 = Number To Fractional String(number=w656) -> (F-format string=w662:string)  [unwired: 3 in]
              n138 = Concatenate Strings(", 90, External, Play_Audio_Tone_Match," ("text"), w662) -> (w660:string)
              n139 = call "write-log.vi"("Write Text"=w660, "Internal Cluster"=w664) -> ()  [unwired: 10 in]
            }
            frame 1 {
              # "Duration (ms)"
              # "Amplitude (V)"
              # "Match"
              n140 = Unbundle By Name(w669) -> ("Tone 2"=w665:i32)
              n141 = control-ref of="Speaker"() -> (w666:refnum<vi>)
              n142 = call-poly "Device.vi"("Amplitude (V)"=5.0, "Device reference"=w666, "Duration (ms)"=200.0, "Frequency (Hz)"=w665) -> ()  [unwired: 7 in, 1 out]
              n143 = Number To Fractional String(number=w665) -> (F-format string=w670:string)  [unwired: 3 in]
              n144 = Concatenate Strings(", 90, External, Play_Audio_Tone_Match," ("text"), w670) -> (w671:string)
              n145 = call "write-log.vi"("Write Text"=w671, "Internal Cluster"=w673) -> ()  [unwired: 10 in]
            }
            frame 2 {
              # "Duration (ms)"
              # "Amplitude (V)"
              # "Non-match"
              n146 = Unbundle By Name(w678) -> ("Tone 1"=w674:i32)
              n147 = control-ref of="Speaker"() -> (w675:refnum<vi>)
              n148 = call-poly "Device.vi"("Amplitude (V)"=5.0, "Device reference"=w675, "Duration (ms)"=200.0, "Frequency (Hz)"=w674) -> ()  [unwired: 7 in, 1 out]
              n149 = Number To Fractional String(number=w674) -> (F-format string=w679:string)  [unwired: 3 in]
              n150 = Concatenate Strings(", 89, External, Play_Audio_Tone_Nonmatch," ("text"), w679) -> (w680:string)
              n151 = call "write-log.vi"("Write Text"=w680, "Internal Cluster"=w682) -> ()  [unwired: 10 in]
            }
            frame 3 {
              # "Duration (ms)"
              # "Amplitude (V)"
              # "Non-match"
              n152 = Unbundle By Name(w687) -> ("Tone 2"=w683:i32)
              n153 = control-ref of="Speaker"() -> (w684:refnum<vi>)
              n154 = call-poly "Device.vi"("Amplitude (V)"=5.0, "Device reference"=w684, "Duration (ms)"=200.0, "Frequency (Hz)"=w683) -> ()  [unwired: 7 in, 1 out]
              n155 = Number To Fractional String(number=w683) -> (F-format string=w688:string)  [unwired: 3 in]
              n156 = Concatenate Strings(", 89, External, Play_Audio_Tone_Nonmatch," ("text"), w688) -> (w689:string)
              n157 = call "write-log.vi"("Write Text"=w689, "Internal Cluster"=w691) -> ()  [unwired: 10 in]
            }
          }
          n158 = call-poly "Rack.vi"() -> ("error out"=w644:errorcluster, "Data Cluster"=w642:T1)  [unwired: 10 in]
          n159 = local write "InputData"(w642) -> ()
          n160 = control-ref of="Lickometer"() -> (w643:refnum<vi>)
          n161 = call-poly "Device.vi"("Device reference"=w643, "error in (no error)"=w644) -> ("Lick start?"=w639:bool)  [unwired: 7 in, 2 out]
          n162 = case shown="True" w639 {
            tunnel: w641 -> [w648 w649]
            tunnel: [w648 w653] -> w640
            frame False {
            }
            frame True {
              n163 = Unbundle By Name(w649) -> ("Licks"=w652:i32)
              n164 = Increment(x=w652) -> (x+1=w651:i32)
              n165 = Bundle By Name(cluster=w649, "Licks"=w651) -> (w653:T17)
              n166 = call "write-log.vi"("Write Text"=", 53, Internal, Lick, Speaker-1" ("text"), "Internal Cluster"=w649) -> ()  [unwired: 10 in]
            }
          }
          n167 = node-c288() -> ()  [unwired: 1 in, 1 out]
        }
        n168 = Unbundle By Name(w355) -> ("Min Licks"=w372:i32, "Trial delay (ms)"=w404:dbl, "Trial window (ms)"=w396:dbl)
        n169 = call <vilib>:"High Resolution Relative Seconds.vi"() -> ("relative seconds"=w405:dbl)
        n170 = case shown="3" w351 {
          tunnel: [w731 w735 w739 w743] -> w429
          tunnel: [w730 w734 w738 w742] -> w428
          tunnel: [w729 w733 w737 w741] -> w427
          tunnel: [w728 w732 w736 w740] -> w426
          frame 0, Default {
            w728 = FALSE  # Trial CR
            w729 = FALSE  # Trial FA
            w730 = TRUE  # Trial Miss
            w731 = FALSE  # Trial Hit
            # "Match"
          }
          frame 1 {
            w732 = FALSE  # Trial CR
            w733 = FALSE  # Trial FA
            w734 = TRUE  # Trial Miss
            w735 = FALSE  # Trial Hit
            # "Match"
          }
          frame 2 {
            w736 = TRUE  # Trial CR
            w737 = FALSE  # Trial FA
            w738 = FALSE  # Trial Miss
            w739 = FALSE  # Trial Hit
            # "Nonmatch"
          }
          frame 3 {
            w740 = TRUE  # Trial CR
            w741 = FALSE  # Trial FA
            w742 = FALSE  # Trial Miss
            w743 = FALSE  # Trial Hit
            # "Nonmatch"
          }
        }
        n171 = Add(x=w404, y=w396) -> (x+y=w403:dbl)
        n172 = Bundle("Trial Hit"=w429, "Trial Miss"=w428, "Trial FA"=w427, "Trial CR"=w426, "Skip Receiving"=w376) -> (w425:T21)  [unwired: 1 in]
        n173 = Divide(x=w404, y=1000.0) -> (x/y=w433:dbl)
        n174 = node-c288(w365) -> ()  [unwired: 1 out]
        n175 = node-c288(i64 2 ("Period")) -> (w363:T18)  [unwired: 3 in]
        n176 = timed-loop {
          tunnel: w433 -> [w591]
          tunnel: w405 -> [w606]
          shift-right: [w607] -> w354
          shift-left: w430 -> [w600]
          shift-right: [w604] -> w424
          shift-left: w425 -> [w605]
          tunnel: w372 -> [w596]
          shift-right: [w598] -> _
          shift-left: w374 -> [w599]
          timing: w363 -> [_]
          timing-out: [_] -> w362
          i -> [w603]
          stop <- w601 stop-if-true
          # "Min Lick Counter"
          # "Read licks"
          n177 = node-c288() -> ()  [unwired: 1 in, 1 out]
          n178 = call-poly "Rack.vi"() -> ("error out"=w594:errorcluster, "Data Cluster"=w592:T1)  [unwired: 10 in]
          n179 = control-ref of="Lickometer"() -> (w593:refnum<vi>)
          n180 = local write "InputData"(w592) -> ()
          n181 = call-poly "Device.vi"("Device reference"=w593, "error in (no error)"=w594) -> ("Lick start?"=w595:bool)  [unwired: 7 in, 2 out]
          n182 = case shown="True" w595 {
            tunnel: w599 -> [w611 w613]
            tunnel: [w611 w612] -> w598
            frame False {
            }
            frame True {
              n183 = Increment(x=w613) -> (x+1=w612:i32)
            }
          }
          n184 = Greater Or Equal?(x=w598, y=w596) -> (x >= y?=w597:bool)
          n185 = call <vilib>:"High Resolution Relative Seconds.vi"() -> ("relative seconds"=w608:dbl)
          n186 = Subtract(x=w608, y=w606) -> (x-y=w590:dbl)
          n187 = Subtract(x=w591, y=w590) -> (x-y=w589:dbl)
          n188 = local write "Time"(w589) -> ()
          n189 = case shown="True" w595 {
            tunnel: w600 -> [w627 w629]
            tunnel: [w627 w630] -> w607
            tunnel: w605 -> [w626 w628]
            tunnel: [w626 w628] -> w604
            tunnel: w597 -> [_ _]
            frame False {
            }
            frame True {
              # "Do nothing if licking during delay"
              # "If a lick is received"
              # "Write lick to log"
              n190 = Unbundle By Name(w629) -> ("Licks"=w632:i32)
              n191 = Increment(x=w632) -> (x+1=w631:i32)
              n192 = Bundle By Name(cluster=w629, "Licks"=w631) -> (w630:T17)
              n193 = call "write-log.vi"("Write Text"=", 51, Internal, Lick, Trial_Delay" ("text"), "Internal Cluster"=w629) -> ()  [unwired: 10 in]
            }
          }
          n194 = Greater Or Equal?(x=w590, y=w591) -> (x >= y?=w601:bool)
          n195 = case shown="True" w601 {
            tunnel: w600 -> [_ w615]
            frame False {
            }
            frame True {
              # "Exit Log"
              n196 = call "write-log.vi"("Write Text"=", 93, Internal, End_Trial_Delay_Window, " ("text"), "Internal Cluster"=w615) -> ()  [unwired: 10 in]
            }
          }
          n197 = Equal To 0?(x=w603) -> (x = 0?=w602:bool)
          n198 = case shown="True" w602 {
            tunnel: w600 -> [_ w616]
            tunnel: w591 -> [_ w617]
            frame False {
            }
            frame True {
              n199 = stacked-sequence {
                tunnel: w617 -> [_ w621]
                tunnel: w616 -> [w619 w622]
                frame #0 {
                  n200 = Unbundle By Name(w619) -> ("Next Trial"=w620:i32)
                  n201 = Equal To 0?(x=w620) -> (x = 0?=w618:bool)
                  n202 = case shown="False" w618 {
                    tunnel: w619 -> [_ _]
                    frame False {
                      # "CS+"
                    }
                    frame True {
                      # "CS-"
                    }
                  }
                }
                frame #1 {
                  n203 = Number To Fractional String(number=w621) -> (F-format string=w623:string)  [unwired: 3 in]
                  n204 = Concatenate Strings(", 91, Internal, Start_Trial_Delay_Window, " ("text"), w623) -> (w624:string)
                  n205 = call "write-log.vi"("Write Text"=w624, "Internal Cluster"=w622) -> ()  [unwired: 10 in]
                }
              }
            }
          }
          n206 = node-c288() -> ()  [unwired: 1 in, 1 out]
        }
        n207 = Unbundle By Name(w355) -> ("Reward Vol. (uL)"=w369:dbl)
        n208 = node-c288(w362) -> ()  [unwired: 1 out]
        n209 = node-c288() -> (w357:T18)  [unwired: 4 in]
        n210 = timed-loop {
          tunnel: w354 -> [w445]
          tunnel: [w441] -> w353
          tunnel: w355 -> [w444]
          timing: w357 -> [_]
          timing-out: [_] -> w356
          stop <- TRUE stop-if-true
          # "Read Speaker Lick"
          # "Play Sound While Loop"
          n211 = node-c288() -> ()  [unwired: 1 in, 1 out]
          n212 = Unbundle By Name(w445) -> ("Next Trial"=w439:i32)
          n213 = case shown="3" w439 {
            tunnel: w445 -> [w463 w472 w481 w490]
            tunnel: [w463 w472 w481 w490] -> w442
            tunnel: w444 -> [w462 w468 w477 w486]
            frame 0, Default {
              # "Duration (ms)"
              # "Amplitude (V)"
              # "Match"
              n214 = Unbundle By Name(w462) -> ("Tone 1"=w456:i32)
              n215 = control-ref of="Speaker"() -> (w455:refnum<vi>)
              n216 = call-poly "Device.vi"("Amplitude (V)"=5.0, "Device reference"=w455, "Duration (ms)"=200.0, "Frequency (Hz)"=w456) -> ()  [unwired: 7 in, 1 out]
              n217 = Number To Fractional String(number=w456) -> (F-format string=w461:string)  [unwired: 3 in]
              n218 = Concatenate Strings(", 90, External, Play_Audio_Tone_Match," ("text"), w461) -> (w459:string)
              n219 = call "write-log.vi"("Write Text"=w459, "Internal Cluster"=w463) -> ()  [unwired: 10 in]
            }
            frame 1 {
              # "Duration (ms)"
              # "Amplitude (V)"
              # "Match"
              n220 = Unbundle By Name(w468) -> ("Tone 2"=w465:i32)
              n221 = control-ref of="Speaker"() -> (w464:refnum<vi>)
              n222 = call-poly "Device.vi"("Amplitude (V)"=5.0, "Device reference"=w464, "Duration (ms)"=200.0, "Frequency (Hz)"=w465) -> ()  [unwired: 7 in, 1 out]
              n223 = Number To Fractional String(number=w465) -> (F-format string=w469:string)  [unwired: 3 in]
              n224 = Concatenate Strings(", 90, External, Play_Audio_Tone_Match," ("text"), w469) -> (w470:string)
              n225 = call "write-log.vi"("Write Text"=w470, "Internal Cluster"=w472) -> ()  [unwired: 10 in]
            }
            frame 2 {
              # "Duration (ms)"
              # "Amplitude (V)"
              # "Non-match"
              n226 = Unbundle By Name(w477) -> ("Tone 2"=w474:i32)
              n227 = control-ref of="Speaker"() -> (w473:refnum<vi>)
              n228 = call-poly "Device.vi"("Amplitude (V)"=5.0, "Device reference"=w473, "Duration (ms)"=200.0, "Frequency (Hz)"=w474) -> ()  [unwired: 7 in, 1 out]
              n229 = Number To Fractional String(number=w474) -> (F-format string=w478:string)  [unwired: 3 in]
              n230 = Concatenate Strings(", 89, External, Play_Audio_Tone_Nonmatch," ("text"), w478) -> (w479:string)
              n231 = call "write-log.vi"("Write Text"=w479, "Internal Cluster"=w481) -> ()  [unwired: 10 in]
            }
            frame 3 {
              # "Duration (ms)"
              # "Amplitude (V)"
              # "Non-match"
              n232 = Unbundle By Name(w486) -> ("Tone 1"=w483:i32)
              n233 = control-ref of="Speaker"() -> (w482:refnum<vi>)
              n234 = call-poly "Device.vi"("Amplitude (V)"=5.0, "Device reference"=w482, "Duration (ms)"=200.0, "Frequency (Hz)"=w483) -> ()  [unwired: 7 in, 1 out]
              n235 = Number To Fractional String(number=w483) -> (F-format string=w487:string)  [unwired: 3 in]
              n236 = Concatenate Strings(", 89, External, Play_Audio_Tone_Nonmatch," ("text"), w487) -> (w488:string)
              n237 = call "write-log.vi"("Write Text"=w488, "Internal Cluster"=w490) -> ()  [unwired: 10 in]
            }
          }
          n238 = call-poly "Rack.vi"() -> ("error out"=w443:errorcluster, "Data Cluster"=w438:T1)  [unwired: 10 in]
          n239 = local write "InputData"(w438) -> ()
          n240 = control-ref of="Lickometer"() -> (w437:refnum<vi>)
          n241 = call-poly "Device.vi"("Device reference"=w437, "error in (no error)"=w443) -> ("Lick start?"=w440:bool)  [unwired: 7 in, 2 out]
          n242 = case shown="True" w440 {
            tunnel: w442 -> [w447 w448]
            tunnel: [w447 w452] -> w441
            frame False {
            }
            frame True {
              n243 = Unbundle By Name(w448) -> ("Licks"=w451:i32)
              n244 = Increment(x=w451) -> (x+1=w450:i32)
              n245 = Bundle By Name(cluster=w448, "Licks"=w450) -> (w452:T17)
              n246 = call "write-log.vi"("Write Text"=", 53, Internal, Lick, Speaker-2" ("text"), "Internal Cluster"=w448) -> ()  [unwired: 10 in]
            }
          }
          n247 = node-c288() -> ()  [unwired: 1 in, 1 out]
        }
        n248 = node-c288(w356) -> ()  [unwired: 1 out]
        n249 = node-c288(i64 2 ("Period")) -> (w360:T18)  [unwired: 3 in]
        n250 = Divide(x=w403, y=1000.0) -> (x/y=w432:dbl)
        n251 = Divide(x=w396, y=1000.0) -> (x/y=w397:dbl)
        n252 = timed-loop {
          tunnel: w432 -> [w495]
          tunnel: w405 -> [w511]
          shift-right: [w512] -> w375
          shift-left: w353 -> [w504]
          tunnel: w397 -> [w506]
          shift-right: [w509] -> w395
          shift-left: w424 -> [w510]
          shift-right: [w502] -> _
          shift-left: w373 -> [w503]
          tunnel: w372 -> [w501]
          timing: w360 -> [_]
          timing-out: [_] -> w359
          i -> [w508]
          stop <- w505 stop-if-true
          # "Min Lick Counter"
          # "Read licks"
          n253 = node-c288() -> ()  [unwired: 1 in, 1 out]
          n254 = control-ref of="Lickometer"() -> (w497:refnum<vi>)
          n255 = call-poly "Rack.vi"() -> ("error out"=w499:errorcluster, "Data Cluster"=→"InputData":T1)  [unwired: 10 in]
          n256 = call-poly "Device.vi"("Device reference"=w497, "error in (no error)"=w499) -> ("Lick start?"=w498:bool)  [unwired: 7 in, 2 out]
          n257 = case shown="False" w498 {
            tunnel: w503 -> [w516 w518]
            tunnel: [w516 w517] -> w502
            frame False {
            }
            frame True {
              n258 = Increment(x=w518) -> (x+1=w517:i32)
            }
          }
          n259 = call <vilib>:"High Resolution Relative Seconds.vi"() -> ("relative seconds"=w513:dbl)
          n260 = Greater Or Equal?(x=w502, y=w501) -> (x >= y?=w500:bool)
          n261 = Subtract(x=w513, y=w511) -> (x-y=w494:dbl)
          n262 = Subtract(x=w495, y=w494) -> (x-y=w493:dbl)
          n263 = local write "Time"(w493) -> ()
          n264 = Greater Or Equal?(x=w494, y=w495) -> (x >= y?=w505:bool)
          n265 = case shown="True" w505 {
            tunnel: w504 -> [_ w519]
            frame False {
            }
            frame True {
              # "Exit Log"
              n266 = stacked-sequence {
                tunnel: w519 -> [w520 w524]
                frame #0 {
                  n267 = call "write-log.vi"("Write Text"=", 94, Internal, End_Trial_Reception_Window, " ("text"), "Internal Cluster"=w520) -> ()  [unwired: 10 in]
                }
                frame #1 {
                  n268 = Unbundle By Name(w524) -> ("Next Trial"=w523:i32)
                  n269 = Equal To 0?(x=w523) -> (x = 0?=w522:bool)
                  n270 = case shown="True" w522 {
                    tunnel: w524 -> [_ _]
                    frame False {
                    }
                    frame True {
                    }
                  }
                }
              }
            }
          }
          n271 = Equal To 0?(x=w508) -> (x = 0?=w507:bool)
          n272 = case shown="True" w498 {
            tunnel: w504 -> [w531 w535]
            tunnel: [w531 w536] -> w512
            tunnel: w510 -> [w530 w534]
            tunnel: [w530 w533] -> w509
            tunnel: w500 -> [_ w532]
            frame False {
            }
            frame True {
              # "Write lick to log"
              n273 = case shown="True" w532 {
                tunnel: w535 -> [_ w544]
                tunnel: w534 -> [w540 w543]
                tunnel: [w540 w542] -> w533
                frame False {
                }
                frame True {
                  n274 = Unbundle By Name(w544) -> ("Next Trial"=w541:i32)
                  n275 = case shown="3" w541 {
                    tunnel: w543 -> [w546 w556 w566 w576]
                    tunnel: [w545 w555 w565 w575] -> w542
                    frame 0, Default {
                      # "Match"
                      n276 = Unbundle By Name(w546) -> ("Skip Receiving"=w547:bool)
                      n277 = case shown="False" w547 {
                        tunnel: w546 -> [w549 w554]
                        tunnel: [w548 w554] -> w545
                        frame False {
                          n278 = Bundle By Name(cluster=w549, "Trial Hit"=TRUE, "Trial Miss"=FALSE, "Trial FA"=FALSE ("Trial CR"), "Trial CR"=FALSE ("Trial FA")) -> (w548:T21)
                        }
                        frame True {
                        }
                      }
                    }
                    frame 1 {
                      # "Match"
                      n279 = Unbundle By Name(w556) -> ("Skip Receiving"=w557:bool)
                      n280 = case shown="False" w557 {
                        tunnel: w556 -> [w559 w564]
                        tunnel: [w558 w564] -> w555
                        frame False {
                          n281 = Bundle By Name(cluster=w559, "Trial Hit"=TRUE, "Trial Miss"=FALSE, "Trial FA"=FALSE ("Trial CR"), "Trial CR"=FALSE ("Trial FA")) -> (w558:T21)
                        }
                        frame True {
                        }
                      }
                    }
                    frame 2 {
                      # "Non-match"
                      n282 = Unbundle By Name(w566) -> ("Skip Receiving"=w567:bool)
                      n283 = case shown="False" w567 {
                        tunnel: w566 -> [w569 w574]
                        tunnel: [w568 w574] -> w565
                        frame False {
                          n284 = Bundle By Name(cluster=w569, "Trial Hit"=FALSE, "Trial Miss"=FALSE, "Trial FA"=TRUE ("Trial CR"), "Trial CR"=FALSE ("Trial FA")) -> (w568:T21)
                        }
                        frame True {
                        }
                      }
                    }
                    frame 3 {
                      # "Non-match"
                      n285 = Unbundle By Name(w576) -> ("Skip Receiving"=w577:bool)
                      n286 = case shown="False" w577 {
                        tunnel: w576 -> [w579 w584]
                        tunnel: [w578 w584] -> w575
                        frame False {
                          n287 = Bundle By Name(cluster=w579, "Trial Hit"=FALSE, "Trial Miss"=FALSE, "Trial FA"=TRUE ("Trial CR"), "Trial CR"=FALSE ("Trial FA")) -> (w578:T21)
                        }
                        frame True {
                        }
                      }
                    }
                  }
                }
              }
              n288 = Unbundle By Name(w535) -> ("Licks"=w538:i32)
              n289 = Increment(x=w538) -> (x+1=w537:i32)
              n290 = Bundle By Name(cluster=w535, "Licks"=w537) -> (w536:T17)
              n291 = call "write-log.vi"("Write Text"=", 52, Internal, Lick, Trial_Reception_Window" ("text"), "Internal Cluster"=w535) -> ()  [unwired: 10 in]
            }
          }
          n292 = case shown="True" w507 {
            tunnel: w504 -> [_ w529]
            tunnel: w506 -> [_ w525]
            frame False {
            }
            frame True {
              n293 = Number To Fractional String(number=w525) -> (F-format string=w526:string)  [unwired: 3 in]
              n294 = Concatenate Strings(", 92, Internal, Start_Trial_Reception_Window, " ("text"), w526) -> (w528:string)
              n295 = call "write-log.vi"("Write Text"=w528, "Internal Cluster"=w529) -> ()  [unwired: 10 in]
            }
          }
          n296 = node-c288() -> ()  [unwired: 1 in, 1 out]
        }
        n297 = Unbundle By Name(w395) -> ("Trial Hit"=w352:bool, "Trial Miss"=w408:bool, "Trial FA"=w407:bool, "Trial CR"=w406:bool)
        n298 = case shown="True" w352 {
          tunnel: w375 -> [w717 w725]
          tunnel: [w717 w724] -> w367
          tunnel: w369 -> [_ w720]
          frame False {
          }
          frame True {
            n299 = Unbundle By Name(w725) -> ("Reward Dispensed"=w727:dbl)
            n300 = Add(x=w727, y=w720) -> (x+y=w726:dbl)
            n301 = Bundle By Name(cluster=w725, "Reward Dispensed"=w726) -> (w724:T17)
            n302 = Number To Fractional String(number=w720) -> (F-format string=w721:string)  [unwired: 3 in]
            n303 = Concatenate Strings(", 100, External, Dispense_Reward," ("text"), w721) -> (w723:string)
            n304 = call "write-log.vi"("Write Text"=w723, "Internal Cluster"=w725) -> ()  [unwired: 10 in]
            n305 = control-ref of="Valve"() -> (w719:refnum<vi>)
            n306 = call-poly "Device.vi"("Device reference"=w719, "Duration"=0) -> ()  [unwired: 8 in, 2 out]
          }
        }
        n307 = Or(x=w408, y=w407) -> (x .or. y?=w401:bool)
        n308 = Unbundle By Name(w367) -> ("Hits"=w423:i32, "Miss"=w422:i32, "False Alarm"=w417:i32, "Correct Rejection"=w421:i32)
        n309 = Boolean To (0,1)(Boolean=w352) -> (0, 1=w418:i16)
        n310 = Boolean To (0,1)(Boolean=w408) -> (0, 1=w419:i16)
        n311 = Boolean To (0,1)(Boolean=w407) -> (0, 1=w416:i16)
        n312 = Boolean To (0,1)(Boolean=w406) -> (0, 1=w420:i16)
        n313 = Add(x=w418, y=w423) -> (x+y=w413:i32)
        n314 = Add(x=w416, y=w417) -> (x+y=w415:i32)
        n315 = Add(x=w419, y=w422) -> (x+y=w414:i32)
        n316 = Add(x=w420, y=w421) -> (x+y=w412:i32)
        n317 = Compound Arithmetic op=ADD(w413, w412) -> (w411:i32)
        n318 = Compound Arithmetic op=ADD(w413, w414, w415, w412) -> (w410:i32)
        n319 = Divide(x=w411, y=w410) -> (x/y=w409:dbl)
        n320 = Unbundle By Name(w395) -> ("Trial Hit"=w394:bool, "Trial Miss"=w385:bool, "Trial FA"=w384:bool, "Trial CR"=w383:bool)
        n321 = Bundle By Name(cluster=w367, "Hits"=w413, "Miss"=w414, "False Alarm"=w415, "Correct Rejection"=w412, "Accuracy"=w409, "Punish ITI"=w401) -> (w377:T17)
        n322 = Select(t=", 62, Internal, Trial_FA," ("text"), s=w384, f="") -> (s? t:f=w380:string)
        n323 = Select(t=", 60, Internal, Trial_Hit," ("text"), s=w394, f="") -> (s? t:f=w382:string)
        n324 = Select(t=", 61, Internal, Trial_Miss," ("text"), s=w385, f="") -> (s? t:f=w381:string)
        n325 = Select(t=", 63, Internal, Trial_CR," ("text"), s=w383, f="") -> (s? t:f=w379:string)
        n326 = Concatenate Strings(w382, w381, w380, w379) -> (w378:string)
        n327 = stacked-sequence {
          tunnel: w378 -> [w697 _]
          tunnel: w377 -> [w696 w700]
          tunnel: [_ w699] -> w368
          tunnel: [_ w698] -> _
          tunnel: w351 -> [_ w698]
          frame #0 {
            # "Trial_"
            n328 = call "write-log.vi"("Write Text"=w697, "Internal Cluster"=w696) -> ()  [unwired: 10 in]
          }
          frame #1 {
            n329 = case shown="3" w698 {
              tunnel: w700 -> [w701 w703 w705 w707]
              tunnel: [w701 w703 w705 w707] -> w699
              frame 0, Default {
                n330 = call "write-log.vi"("Write Text"=", 97, Internal, End_Match_Trial, " ("text"), "Internal Cluster"=w701) -> ()  [unwired: 10 in]
              }
              frame 1 {
                n331 = call "write-log.vi"("Write Text"=", 97, Internal, End_Match_Trial, " ("text"), "Internal Cluster"=w703) -> ()  [unwired: 10 in]
              }
              frame 2 {
                n332 = call "write-log.vi"("Write Text"=", 98, Internal, End_Nonmatch_Trial, " ("text"), "Internal Cluster"=w705) -> ()  [unwired: 10 in]
              }
              frame 3 {
                n333 = call "write-log.vi"("Write Text"=", 98, Internal, End_Nonmatch_Trial, " ("text"), "Internal Cluster"=w707) -> ()  [unwired: 10 in]
              }
            }
          }
        }
        n334 = node-c288(w359) -> ()  [unwired: 1 out]
        n335 = Select(t="Punish ITI", s=w401, f="ITI") -> (s? t:f=w402:string)
      }
      frame "Stop" {
        n336 = call "write-log.vi"("Write Text"=", 110, External, End_Session_Trials_Finished, " ("text"), "Internal Cluster"=w745) -> ()  [unwired: 10 in]
      }
    }
    "Current State" <- w268
    n337 = Unbundle By Name(w246) -> ("relative seconds"=w273:dbl)
    n338 = Unbundle By Name(w267) -> ("Max Time (s)"=w272:dbl)
    n339 = call <vilib>:"High Resolution Relative Seconds.vi"() -> ("relative seconds"=w274:dbl)
    n340 = Subtract(x=w274, y=w273) -> (x-y=w270:dbl)
    "Time Elapsed" <- w270
    n341 = Greater Or Equal?(x=w270, y=w272) -> (x >= y?=w244:bool)
    n342 = Or(x="stop", y=w244) -> (x .or. y?=w242:bool)
    n343 = Or(x=w271, y=w242) -> (x .or. y?=w247:bool)
    n344 = case shown="True" w242 {
      tunnel: w246 -> [_ w276]
      frame False {
      }
      frame True {
        n345 = call "write-log.vi"("Write Text"=", 111, External, End_Session_Time_Reached, " ("text"), "Internal Cluster"=w276) -> ()  [unwired: 10 in]
      }
    }
    n346 = Unbundle By Name(w266) -> ("Accuracy"=→"Acc":dbl, "Hits"=w253:i32, "Miss"=w254:i32, "False Alarm"=w255:i32, "Correct Rejection"=w256:i32, "Current Trial Index"=w249:i32, "Licks"=w257:i32, "Reward Dispensed"=w258:dbl)
    n347 = Number To Decimal String(number=w257) -> (decimal integer string=→"Licks":string)  [unwired: 1 in]
    n348 = Number To Fractional String(number=w258) -> (F-format string=→"Reward Dispensed (uL)":string)  [unwired: 3 in]
    n349 = Decrement(x=w249) -> (x-1=w250:i32)
    n350 = Number To Decimal String(number=w253) -> (decimal integer string=→"Hits":string)  [unwired: 1 in]
    n351 = Number To Decimal String(number=w254) -> (decimal integer string=→"Miss":string)  [unwired: 1 in]
    n352 = Number To Decimal String(number=w255) -> (decimal integer string=→"FA":string)  [unwired: 1 in]
    n353 = Number To Decimal String(number=w256) -> (decimal integer string=→"CR":string)  [unwired: 1 in]
    n354 = Number To Decimal String(number=w250) -> (decimal integer string=→"Trials":string)  [unwired: 1 in]
  }
  n355 = Concatenate Strings(w110, w109, w108, w107, w106, w105, w48, w42, w30, w29) -> (w102:string)
  n356 = Write to Text File(file (use dialog)=w104, text=w102) -> (refnum out=w103:refnum<file>)  [unwired: 2 in, 2 out]
  n357 = Concatenate Strings("Match_Delay_Lick,NA\nMatch_Reception_Lick,Hit\nMatch_No_Lick,Miss\nNonmatch_Delay_Lick,NA\nNonmatch_Reception_Lick,False_Alarm\nNonmatch_No_Lick,Correct_Reject", "\r\n") -> (w138:string)
  n358 = Write to Text File(file (use dialog)=w103, text=w138) -> (refnum out=w139:refnum<file>)  [unwired: 2 in, 2 out]
  n359 = Concatenate Strings("Trial_Sequence," ("string"), w140, "\r\n") -> (w172:string)
  n360 = Write to Text File(file (use dialog)=w139, text=w172) -> (refnum out=w173:refnum<file>)  [unwired: 2 in, 2 out]
  n361 = Write to Text File(file (use dialog)=w173, text="\r\n") -> (refnum out=w179:refnum<file>)  [unwired: 2 in, 2 out]
  n362 = Concatenate Strings("----------" ("string"), "\r\n") -> (w178:string)
  n363 = Write to Text File(file (use dialog)=w179, text=w178) -> (refnum out=w145:refnum<file>)  [unwired: 2 in, 2 out]
  n364 = Concatenate Strings("Time, ID, Type, Name, Value" ("string"), "\r\n") -> (w143:string)
  n365 = Write to Text File(file (use dialog)=w145, text=w143) -> (refnum out=w144:refnum<file>)  [unwired: 2 in, 2 out]
  n366 = Close File(refnum=w144) -> ()  [unwired: 1 in, 2 out]
  n367 = Unbundle By Name(w60) -> ("appended path"=w55:path, "Accuracy"=w95:dbl, "Hits"=w94:i32, "Miss"=w93:i32, "False Alarm"=w92:i32, "Correct Rejection"=w91:i32, "Licks"=w90:i32, "Reward Dispensed"=w89:dbl)
  n368 = control-ref of="Lickometer"() -> (w22:refnum<vi>)
  n369 = call-poly "Rack.vi"("OutputRequest channel"=w20) -> ("error out"=w24:errorcluster)  [unwired: 10 in]
  n370 = call-poly "Device.vi"("Device reference"=w22, "error in (no error)"=w24) -> ()  [unwired: 9 in, 1 out]
  n371 = Number To Decimal String(number=w90) -> (decimal integer string=w77:string)  [unwired: 1 in]
  n372 = Number To Decimal String(number=w89) -> (decimal integer string=w75:string)  [unwired: 1 in]
  n373 = Number To Decimal String(number=w91) -> (decimal integer string=w79:string)  [unwired: 1 in]
  n374 = Number To Decimal String(number=w93) -> (decimal integer string=w83:string)  [unwired: 1 in]
  n375 = Number To Decimal String(number=w92) -> (decimal integer string=w81:string)  [unwired: 1 in]
  n376 = Number To Decimal String(number=w94) -> (decimal integer string=w85:string)  [unwired: 1 in]
  n377 = Number To Fractional String(number=w95) -> (F-format string=w88:string)  [unwired: 3 in]
  n378 = Concatenate Strings("-1, 120, External, End_Session_Accuracy, " ("text"), w88, "\r\n") -> (w67:string)
  n379 = Concatenate Strings("-1, 125, External, End_Session_Number_Licks, " ("text"), w77, "\r\n") -> (w62:string)
  n380 = Concatenate Strings("-1, 126, External, End_Session_Reward_Dispensed_ml, " ("text"), w75, "\r\n") -> (w61:string)
  n381 = Concatenate Strings("-1, 124, External, End_Session_Number_CR, " ("text"), w79, "\r\n") -> (w63:string)
  n382 = Concatenate Strings("-1, 121, External, End_Session_Number_Hits, " ("text"), w85, "\r\n") -> (w66:string)
  n383 = Concatenate Strings("-1, 122, External, End_Session_Number_Miss, " ("text"), w83, "\r\n") -> (w65:string)
  n384 = Concatenate Strings("-1, 123, External, End_Session_Number_FA, " ("text"), w81, "\r\n") -> (w64:string)
  n385 = Concatenate Strings(w67, w66, w65, w64, w63, w62, w61) -> (w54:string)
  n386 = Open/Create/Replace File(file path (use dialog)=w55) -> (refnum out=w57:refnum<file>)  [unwired: 5 in, 2 out]
  n387 = Set File Position(refnum=w57, from (0:start)=enum16{"start", "end", "current"}."end") -> (refnum out=w59:refnum<file>)  [unwired: 2 in, 1 out]
  n388 = Write to Text File(file (use dialog)=w59, text=w54) -> (refnum out=w56:refnum<file>)  [unwired: 2 in, 2 out]
  n389 = Close File(refnum=w56) -> ()  [unwired: 1 in, 2 out]
